vi "Escape String.vi"(11 "value":string) -> (3 "escaped string":string)   [LabVIEW 2017, in "LVJSON.lvlib" / "JSON String.lvclass"]
uses:
  JSON String.lvclass
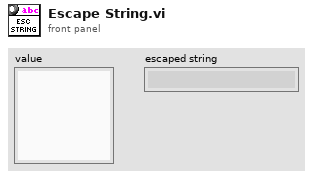
[diagram p1: front panel]
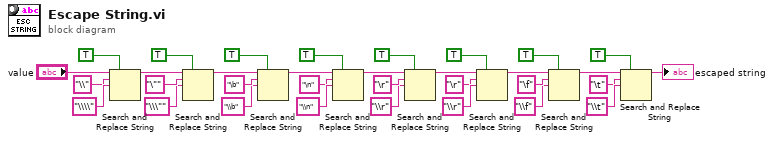
[diagram p0: block diagram]
diagram:
  n1 = Search and Replace String(replace all?=TRUE ("replace all? (F)"), input string="value", search string="\\", replace string="\\\\" ("replace string (\"\")")) -> (result string=w2:string)  [unwired: 4 in, 3 out]
  n2 = Search and Replace String(replace all?=TRUE ("replace all? (F)"), input string=w2, search string="\"", replace string="\\\"" ("replace string (\"\")")) -> (result string=w1:string)  [unwired: 4 in, 3 out]
  n3 = Search and Replace String(replace all?=TRUE ("replace all? (F)"), input string=w1, search string="\b", replace string="\\b" ("replace string (\"\")")) -> (result string=w24:string)  [unwired: 4 in, 3 out]
  n4 = Search and Replace String(replace all?=TRUE ("replace all? (F)"), input string=w24, search string="\n", replace string="\\n" ("replace string (\"\")")) -> (result string=w20:string)  [unwired: 4 in, 3 out]
  n5 = Search and Replace String(replace all?=TRUE ("replace all? (F)"), input string=w20, search string="\r", replace string="\\r" ("replace string (\"\")")) -> (result string=w16:string)  [unwired: 4 in, 3 out]
  n6 = Search and Replace String(replace all?=TRUE ("replace all? (F)"), input string=w16, search string="\r", replace string="\\r" ("replace string (\"\")")) -> (result string=w9:string)  [unwired: 4 in, 3 out]
  n7 = Search and Replace String(replace all?=TRUE ("replace all? (F)"), input string=w9, search string="\f", replace string="\\f" ("replace string (\"\")")) -> (result string=w5:string)  [unwired: 4 in, 3 out]
  n8 = Search and Replace String(replace all?=TRUE ("replace all? (F)"), input string=w5, search string="\t", replace string="\\t" ("replace string (\"\")")) -> (result string=→"escaped string":string)  [unwired: 4 in, 3 out]
